vi "VNA - Initiate and Fetch - Dual Site Parallel_ERMod.vi"(0 "Channel Lists In":string[](array[string]), 5 "Instrument Sessions In":refnum<k15>[](array[refnum]), 7 "VNAs Measurement Parameters":T1, 11 "error in (no error)":errorcluster) -> (4 "Channel Lists Out":string[](array[string]), 6 "Instrument Sessions Out":refnum<k15>[](array[refnum]), 8 "Multisite Cap Data":dbl[][](array[numeric]), 13 "Port 1 Capacitance":dbl[][](array[numeric]), 14 "Port 2 Capacitance":dbl[][](array[numeric]), 15 "error out":errorcluster)   [LabVIEW 2013]
doc: "Initiates and fetches niVNA S11 measurements and converts it to a capacitance measurement."
uses:
  VNAs Measurement Parameters.ctl
  <instrlib>/niVNA/niVNA.llb/niVNA Fetch Receiver Measurement Complex (CDB).vi
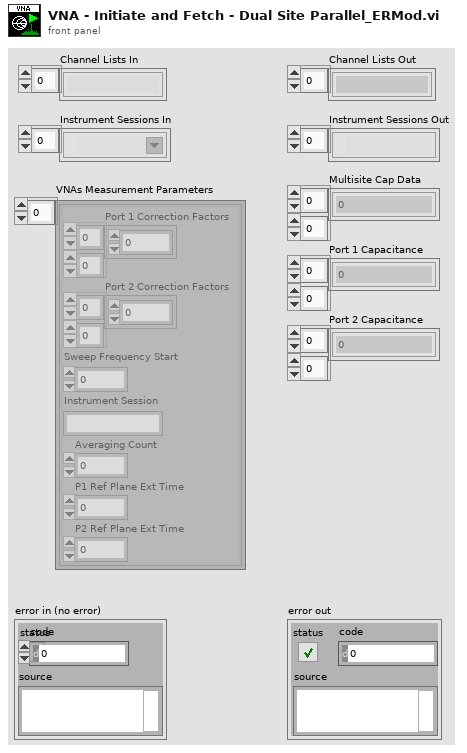
[diagram p1: front panel]
types:
  T1 = typedef "VNAs Measurement Parameters.ctl" = cluster{"Port 1 Correction Factors":cdb[][], "Port 2 Correction Factors":cdb[][], "Sweep Frequency Start":dbl, "Instrument Session":string, "Averaging Count":i32, "P1 Ref Plane Ext Time":dbl, "P2 Ref Plane Ext Time":dbl}[]
  T2 = cluster{"Port 1 Correction Factors":cdb[][], "Port 2 Correction Factors":cdb[][], "Sweep Frequency Start":dbl, "Instrument Session":string, "Averaging Count":i32, "P1 Ref Plane Ext Time":dbl, "P2 Ref Plane Ext Time":dbl}
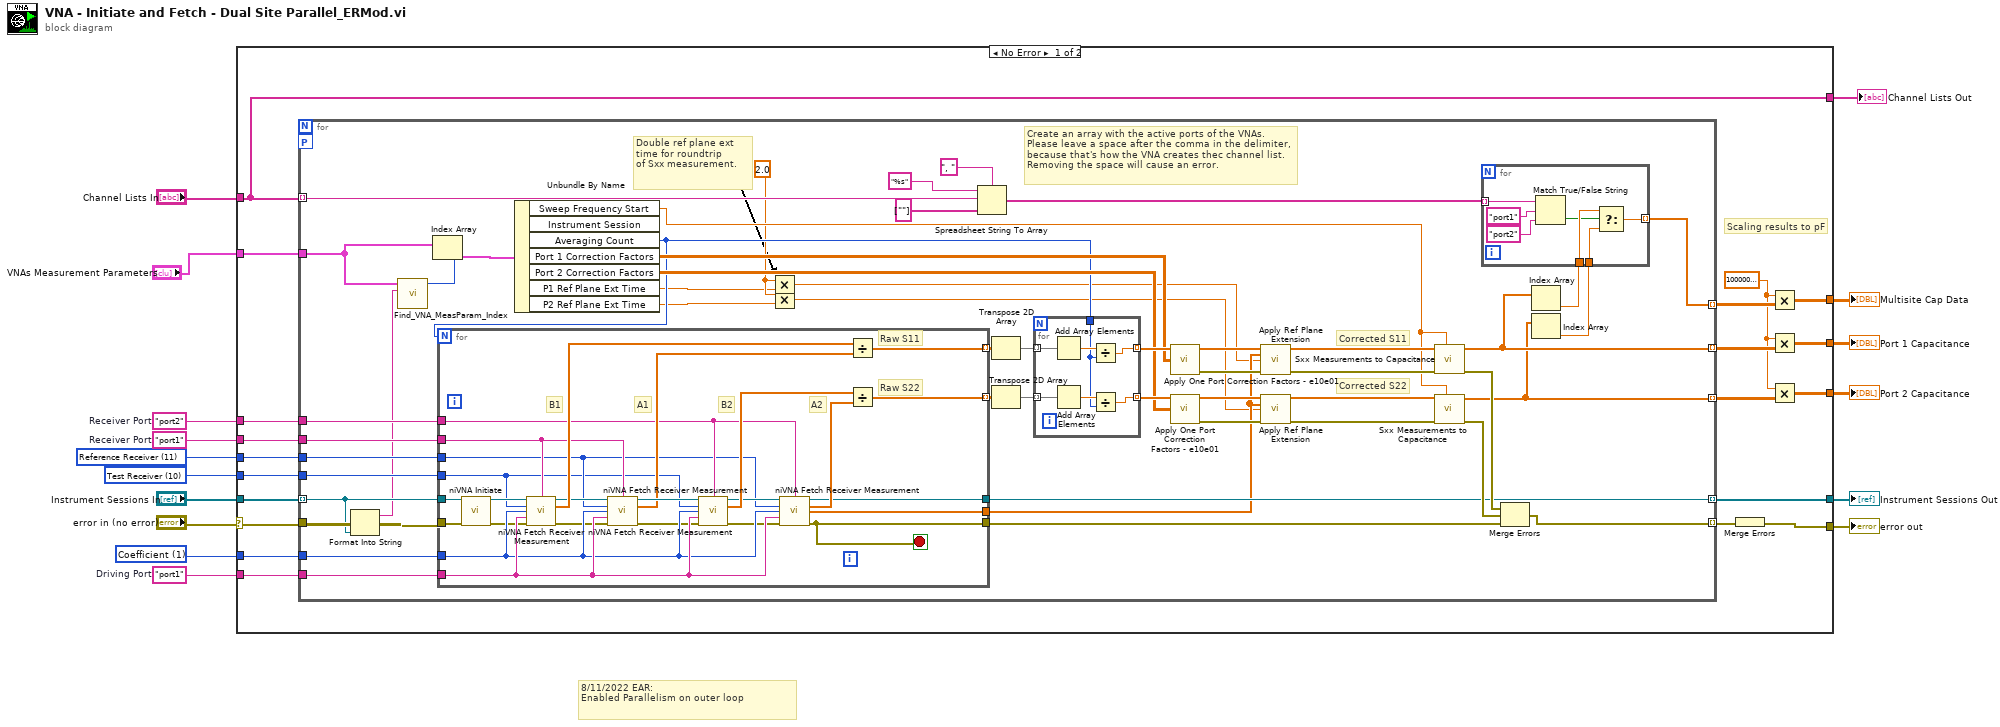
[diagram p0: block diagram]
diagram:
  w5 = 1 items=["Impedance", "Coefficient"] ("format")
  w13 = "port2"  # Receiver Port
  w10 = 10 items=["Test Receiver"=10, "Reference Receiver"=11] ("receiver")
  w9 = "port1"  # Driving Port
  w12 = "port1"  # Receiver Port
  w11 = 11 items=["Test Receiver"=10, "Reference Receiver"=11] ("receiver")
  # "8/11/2022 EAR:\nEnabled Parallelism on outer loop"
  n1 = case shown="No Error" "error in (no error)" {
    selector: "error in (no error)" -> [w18 w130]
    tunnel: [w36 w130] -> w16
    tunnel: [w35 w129] -> w15
    tunnel: "Instrument Sessions In" -> [w34 w129]
    tunnel: w13 -> [w32 _]
    tunnel: w12 -> [w31 _]
    tunnel: w11 -> [w30 _]
    tunnel: w10 -> [w29 _]
    tunnel: w9 -> [w28 _]
    tunnel: [w26 _] -> w8
    tunnel: [w24 _] -> w7
    tunnel: [w22 _] -> w6
    tunnel: w5 -> [w20 _]
    tunnel: "Channel Lists In" -> [w19 w128]
    tunnel: [w19 w128] -> w3
    tunnel: "VNAs Measurement Parameters" -> [w17 _]
    frame No Error {
      w21 = 1000000000000.0 ("x")
      # "Scaling results to pF"
      n2 = for {
        tunnel: w18 -> [w43]
        tunnel: w34 -> [w42] mode=indexing
        tunnel: [w86] -> w33 mode=indexing
        tunnel: [w81] -> w35 mode=indexing
        tunnel: [w56] -> w27 mode=indexing
        tunnel: [w55] -> w25 mode=indexing
        tunnel: w19 -> [w60] mode=indexing
        tunnel: w32 -> [w75]
        tunnel: w31 -> [w74]
        tunnel: w30 -> [w73]
        tunnel: w29 -> [w72]
        tunnel: w20 -> [w71]
        tunnel: w28 -> [w70]
        tunnel: [w54] -> w23 mode=indexing
        tunnel: w17 -> [w41]
        workers-P: _ -> [_]
        w49 = 2.0
        # "Double ref plane ext time for roundtrip\nof Sxx measurement."
        # "Create an array with the active ports of the VNAs.\nPlease leave a space after the comma in the delimiter, \nbecause that's how the VNA creates thec channel list. \nRemoving the space will cause an error."
        # "Corrected S22"
        # "Corrected S11"
        n3 = Format Into String(error in=w43, w42) -> (resulting string=w40:string, error out=w37:errorcluster)  [unwired: 2 in]
        n4 = call "Find_VNA_MeasParam_Index.vi"("Instrument Session"=w40, "VNAs Measurement Parameters"=w41) -> ("Index"=w39:i32)  [unwired: 9 in]
        n5 = Index Array(array=w41, index=w39) -> (element=w44:T2)
        n6 = Unbundle By Name(w44) -> ("Sweep Frequency Start"=w53:dbl, "Averaging Count"=w50:i32, "Port 1 Correction Factors"=w52:cdb[][], "Port 2 Correction Factors"=w51:cdb[][], "P1 Ref Plane Ext Time"=w46:dbl, "P2 Ref Plane Ext Time"=w45:dbl)  [unwired: 1 out]
        n7 = for {
          N: w50 -> [_]
          tunnel: w37 -> [w127]
          tunnel: w42 -> [w126]
          tunnel: [w117] -> w69 mode=indexing
          tunnel: [w116] -> w68 mode=indexing
          tunnel: [w105] -> w38
          tunnel: [w115] -> w81
          tunnel: [w114] -> w76
          tunnel: w75 -> [w113]
          tunnel: w74 -> [w112]
          tunnel: w73 -> [w111]
          tunnel: w72 -> [w110]
          tunnel: w71 -> [w108]
          tunnel: w70 -> [w109]
          stop <- w105 stop-if-true
          # "Raw S22"
          # "Raw S11"
          # "A2"
          # "B2"
          # "B1"
          # "A1"
          n8 = call <instrlib>:"niVNA Initiate.vi"("instrument handle"=w126, "error in"=w127) -> ("instrument handle out"=w118:refnum<k15>, "error out"=w107:errorcluster)  [unwired: 12 in]
          n9 = call-poly <instrlib>:"niVNA Fetch Receiver Measurement.vi"("instrument handle"=w118, "receiver port"=w112, "receiver"=w110, "format"=w108, "driving port"=w109, "error in"=w107) -> ("instrument handle out"=w119:refnum<k15>, "data"=w120:cdb[], "error out"=w106:errorcluster)  [unwired: 6 in, 1 out]
          n10 = call-poly <instrlib>:"niVNA Fetch Receiver Measurement.vi"("instrument handle"=w119, "receiver port"=w112, "receiver"=w111, "format"=w108, "driving port"=w109, "error in"=w106) -> ("instrument handle out"=w123:refnum<k15>, "data"=w121:cdb[], "error out"=w104:errorcluster)  [unwired: 6 in, 1 out]
          n11 = call-poly <instrlib>:"niVNA Fetch Receiver Measurement.vi"("instrument handle"=w123, "receiver port"=w113, "receiver"=w110, "format"=w108, "driving port"=w109, "error in"=w104) -> ("instrument handle out"=w122:refnum<k15>, "data"=w124:cdb[], "error out"=w103:errorcluster)  [unwired: 6 in, 1 out]
          n12 = call-poly <instrlib>:"niVNA Fetch Receiver Measurement.vi"("instrument handle"=w122, "receiver port"=w113, "receiver"=w111, "format"=w108, "driving port"=w109, "error in"=w103) -> ("instrument handle out"=w115:refnum<k15>, "data"=w125:cdb[], "scale points"=w114:dbl[], "error out"=w105:errorcluster)  [unwired: 6 in]
          n13 = Divide(x=w120, y=w121) -> (x/y=w117:cdb[])
          n14 = Divide(x=w124, y=w125) -> (x/y=w116:cdb[])
        }
        n15 = Multiply(x=w49, y=w46) -> (x*y=w48:dbl)
        n16 = Multiply(x=w49, y=w45) -> (x*y=w47:dbl)
        n17 = Spreadsheet String To Array(delimiter (Tab)=", ", format string="%s", spreadsheet string=w60, array type (2D Dbl)=string[] [""]) -> (array=w59:string[])
        n18 = Transpose 2D Array(2D array=w69) -> (transposed array=w67:cdb[][])
        n19 = Transpose 2D Array(2D array=w68) -> (transposed array=w66:cdb[][])
        n20 = for {
          tunnel: w67 -> [w102] mode=indexing
          tunnel: w66 -> [w101] mode=indexing
          tunnel: w50 -> [w98]
          tunnel: [w97] -> w65 mode=indexing
          tunnel: [w96] -> w64 mode=indexing
          n21 = Add Array Elements(numeric array=w102) -> (sum=w100:cdb)
          n22 = Add Array Elements(numeric array=w101) -> (sum=w99:cdb)
          n23 = Divide(x=w100, y=w98) -> (x/y=w97:cdb)
          n24 = Divide(x=w99, y=w98) -> (x/y=w96:cdb)
        }
        n25 = call "Apply One Port Correction Factors - e10e01.vi"("Raw Sxx Data"=w65, "One Port Correction Factors"=w52) -> ("Corrected Sxx Data"=w85:cdb[], "Error Out"=w82:errorcluster)  [unwired: 12 in]
        n26 = call "Apply One Port Correction Factors - e10e01.vi"("Raw Sxx Data"=w64, "One Port Correction Factors"=w51) -> ("Corrected Sxx Data"=w80:cdb[], "Error Out"=w79:errorcluster)  [unwired: 12 in]
        n27 = call "Apply Ref Plane Extension.vi"("Sxx Data"=w85, "Frequencies"=w76, "Ref Plane Extension Time"=w48, "Error In"=w82) -> ("Sxx Data - Ref Plane Shifted"=w84:cdb[], "Error Out"=w83:errorcluster)  [unwired: 10 in]
        n28 = call "Apply Ref Plane Extension.vi"("Sxx Data"=w80, "Frequencies"=w76, "Ref Plane Extension Time"=w47, "Error In"=w79) -> ("Sxx Data - Ref Plane Shifted"=w78:cdb[], "Error Out"=w77:errorcluster)  [unwired: 10 in]
        n29 = call "Sxx Measurements to Capacitance.vi"("Sweep Frequency Start"=w53, "error in (no error)"=w83, "S11 Data"=w84) -> ("error out"=w88:errorcluster, "Capacitance"=w56:dbl[])  [unwired: 7 in]
        n30 = call "Sxx Measurements to Capacitance.vi"("Sweep Frequency Start"=w53, "error in (no error)"=w77, "S11 Data"=w78) -> ("error out"=w87:errorcluster, "Capacitance"=w55:dbl[])  [unwired: 7 in]
        n31 = Merge Errors(w88, w87, w38) -> (w86:errorcluster)
        n32 = Index Array(array=w56) -> (element=w58:dbl)  [unwired: 1 in]
        n33 = Index Array(array=w55) -> (element=w57:dbl)  [unwired: 1 in]
        n34 = for {
          tunnel: w59 -> [w92] mode=indexing
          tunnel: w58 -> [w95]
          tunnel: w57 -> [w94]
          tunnel: [w93] -> w54 mode=indexing
          n35 = Match True/False String(2:"port2", 3:"port1", 4:w92) -> (0:w91:bool)  [unwired: 1 out]
          n36 = Select(t=w95, s=w91, f=w94) -> (s? t:f=w93:dbl)
        }
      }
      n37 = Merge Errors(w33) -> (w36:errorcluster)
      n38 = Multiply(x=w21, y=w23) -> (x*y=w22:dbl[][])
      n39 = Multiply(x=w21, y=w27) -> (x*y=w26:dbl[][])
      n40 = Multiply(x=w21, y=w25) -> (x*y=w24:dbl[][])
    }
    frame Error {
    }
  }
  "error out" <- w16
  "Port 1 Capacitance" <- w8
  "Instrument Sessions Out" <- w15
  "Port 2 Capacitance" <- w7
  "Multisite Cap Data" <- w6
  "Channel Lists Out" <- w3
